vi "_021.vi"() -> ()   [LabVIEW 2024]
panel:
  in  "OK Button":bool
  out "current time":timestamp
  out "iteration":i32
  in  "Stop Button":bool
  out "Gauge":dbl(knob) scale=0.0..10.0
  in  "B":dbl(slide) scale=0.0..10.0
  in  "A":dbl(slide) scale=0.0..10.0
  # "To make a normal oprn with Event Structure :"
  # "To overcome the disadvantages with the help of (Intrept)"
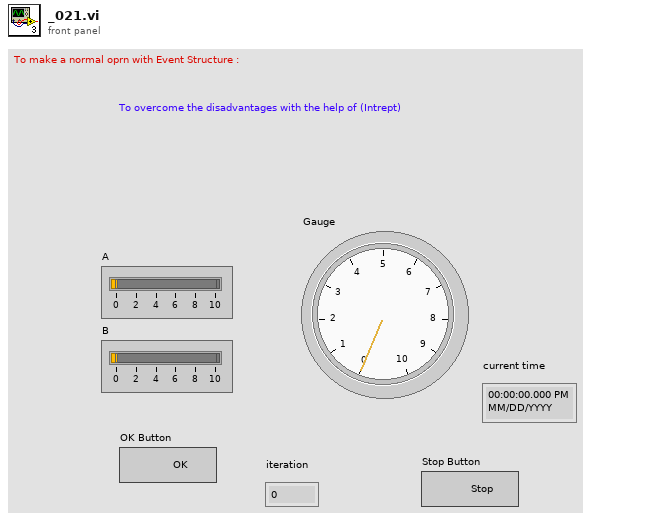
[diagram p1: front panel]
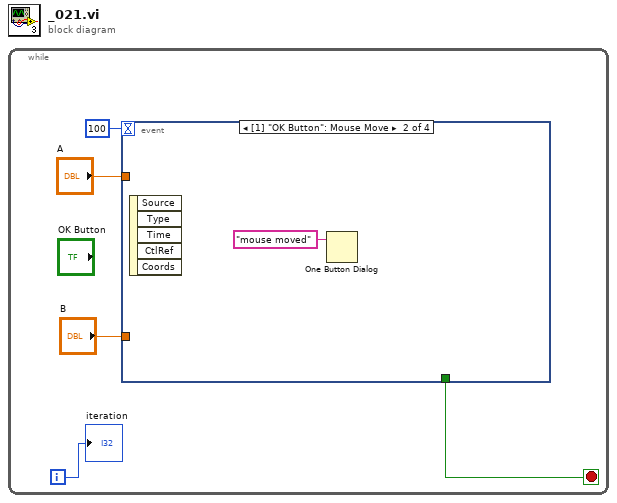
[diagram p0: block diagram]
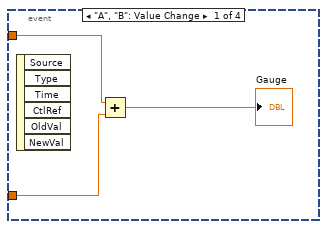
[diagram p2: hidden frame]
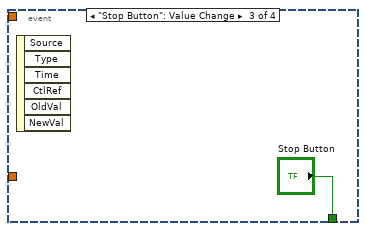
[diagram p3: hidden frame]
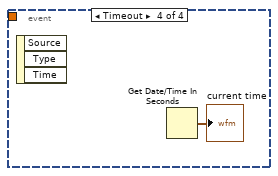
[diagram p4: hidden frame]
diagram:
  n1 = while {
    i -> [w3]
    stop <- w2 stop-if-true
    n2 = event shown="[1] \"OK Button\": Mouse Move" {
      selector: _ -> [_ _ _ _]
      dyn-events: _ -> [_ _ _ _]
      timeout: 100 -> [_ _ _ _]
      tunnel: "B" -> [w8 _ _ _]
      tunnel: "A" -> [w7 _ _ _]
      tunnel: [_ _ "Stop Button" _] -> w2
      event "A", "B": Value Change {
        n3 = event-data() -> ()  [unwired: 1 in, 6 out]
        n4 = Add(x=w7, y=w8) -> (x+y=→"Gauge":dbl)
      }
      event "OK Button": Mouse Move {
        n5 = event-data() -> ()  [unwired: 1 in, 5 out]
        n6 = One Button Dialog(message="mouse moved") -> ()  [unwired: 1 in, 1 out]
      }
      event "Stop Button": Value Change {
        n7 = event-data() -> ()  [unwired: 1 in, 6 out]
      }
      event Timeout {
        n8 = event-data() -> ()  [unwired: 1 in, 3 out]
        n9 = Get Date/Time In Seconds() -> (seconds since 1Jan1904=→"current time":timestamp)
      }
    }
    "iteration" <- w3
  }
